vi "FrequencyCalc.vi"(4 "Checkbox":bool, 6 "Number of teeth in gear":dbl, 7 "Period\n(s) in":dbl, 9 "dt":dbl, 10 "queue in":refnum<queue>, 11 "Queue in":refnum<queue>) -> (0 "Omega [RPM]":dbl(knob) scale=0.0..2000.0, 2 "Period\n(s) out":dbl, 3 "Signal Frequency (Hz)":dbl format="%#_13g", 5 "RPM 2":dbl)   [LabVIEW 2023]
panel:
  out "#Els":dbl
  out "SUM":dbl
  out "Numeric":dbl
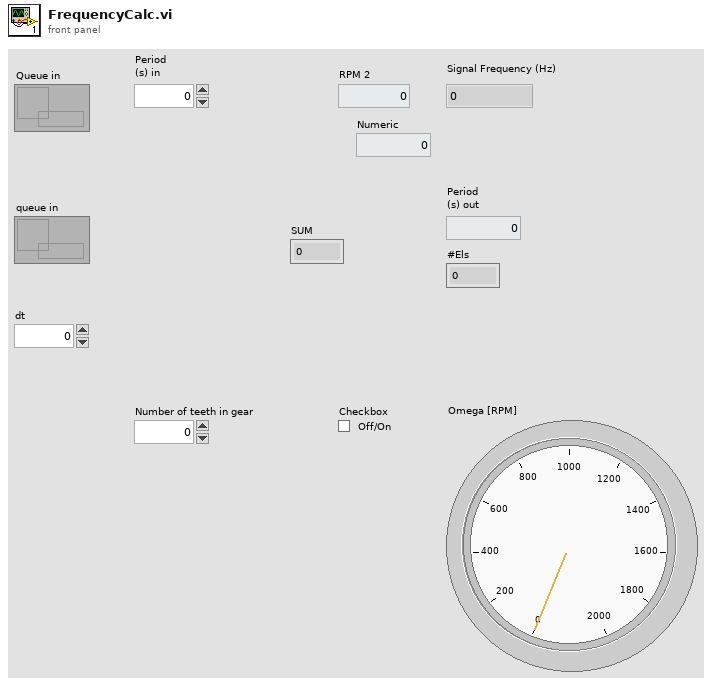
[diagram p1: front panel]
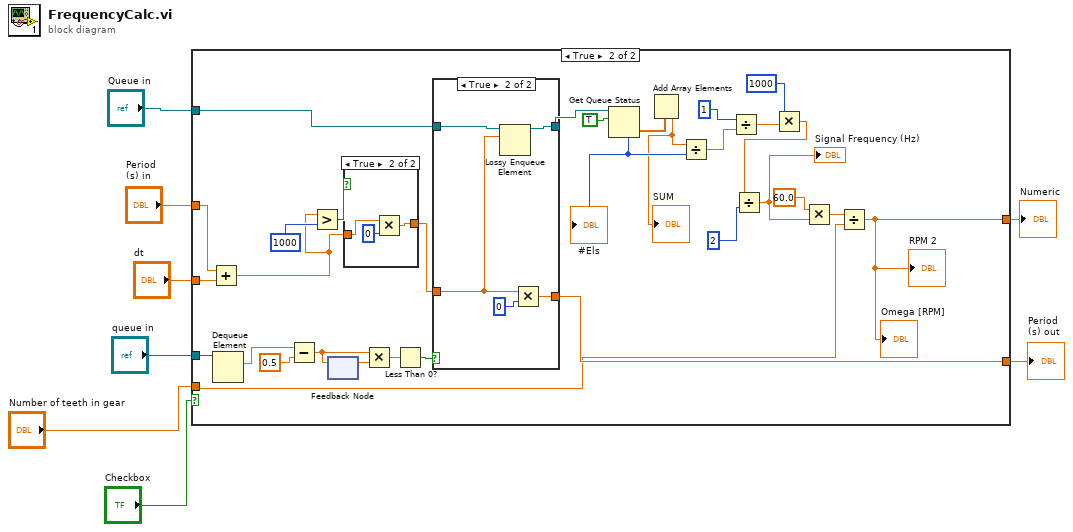
[diagram p0: block diagram]
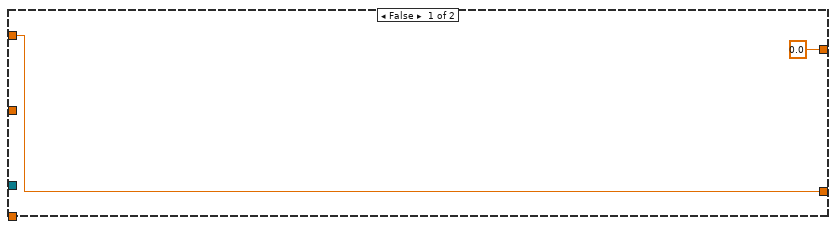
[diagram p2: hidden frame]
diagram:
  n1 = case shown="True" "Checkbox" {
    tunnel: "queue in" -> [_ w41]
    tunnel: "Queue in" -> [_ w35]
    tunnel: "Period\n(s) in" -> [w10 w28]
    tunnel: "dt" -> [_ w27]
    tunnel: [w10 w30] -> w6
    tunnel: "Number of teeth in gear" -> [_ w23]
    tunnel: [0.0 w22] -> w1
    frame False {
    }
    frame True {
      n2 = Add(x=w28, y=w27) -> (x+y=w17:dbl)
      n3 = Dequeue Element(queue=w41) -> (element=w40:dbl)  [unwired: 2 in, 3 out]
      n4 = Subtract(x=w40, y=0.5) -> (x-y=w38:dbl)
      n5 = Greater?(x=w17, y=1000) -> (0:w18:bool)
      n6 = feedback-in #1(w38) -> ()
      n7 = feedback #1() -> (w37:dbl)  [unwired: 1 in]
      n8 = case shown="True" w18 {
        tunnel: w17 -> [w42 w44]
        tunnel: [w42 w43] -> w16
        frame False {
        }
        frame True {
          n9 = Multiply(x=w44, y=0) -> (x*y=w43:dbl)
        }
      }
      n10 = Multiply(x=w38, y=w37) -> (x*y=w36:dbl)
      n11 = Less Than 0?(x=w36) -> (x < 0?=w29:bool)
      n12 = case shown="True" w29 {
        tunnel: w35 -> [w47 w51]
        tunnel: [w47 w50] -> w33
        tunnel: [w46 w49] -> w30
        tunnel: w16 -> [w46 w48]
        frame False {
        }
        frame True {
          n13 = Lossy Enqueue Element(queue=w51, element=w48) -> (queue out=w50:refnum<queue>)  [unwired: 1 in, 3 out]
          n14 = Multiply(x=w48, y=0) -> (x*y=w49:dbl)
        }
      }
      n15 = Get Queue Status(queue=w33, return elements? (F)=TRUE) -> (# elements in queue=w21:i32, elements=w32:dbl[])  [unwired: 1 in, 6 out]
      "#Els" <- w21
      n16 = Add Array Elements(numeric array=w32) -> (sum=w20:dbl)
      "SUM" <- w20
      n17 = Divide(x=w20, y=w21) -> (x/y=w14:dbl)
      n18 = Divide(x=1, y=w14) -> (x/y=w13:dbl)
      n19 = Multiply(x=1000, y=w13) -> (x*y=w11:dbl)
      n20 = Divide(x=w11, y=2) -> (x/y=w25:dbl)
      "Signal Frequency (Hz)" <- w25
      n21 = Multiply(x=60.0, y=w25) -> (x*y=w24:dbl)
      n22 = Divide(x=w24, y=w23) -> (x/y=w22:dbl)
      "RPM 2" <- w22
      "Omega [RPM]" <- w22
    }
  }
  "Period\n(s) out" <- w6
  "Numeric" <- w1
